vi "SFTP Error Status.vi"(8 "error in (no error)":errorcluster, 11 "return value":i32) -> (0 "error out":errorcluster, 3 "return value out":i32)   [LabVIEW 2017, in "libssh2.lvlib"]
uses:
  libssh2.lvlib
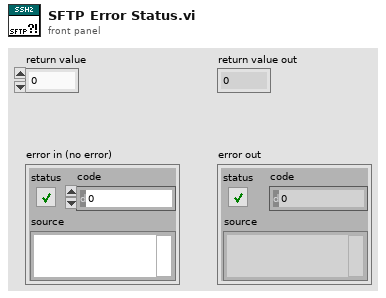
[diagram p1: front panel]
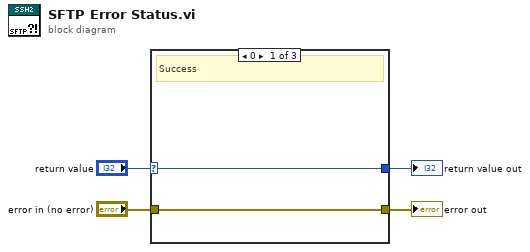
[diagram p0: block diagram]
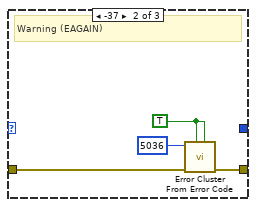
[diagram p2: hidden frame]
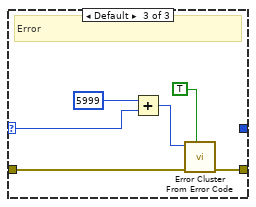
[diagram p3: hidden frame]
diagram:
  n1 = case shown="0" "return value" {
    selector: "return value" -> [w5 _ w11]
    tunnel: "error in (no error)" -> [w6 w10 w15]
    tunnel: [w6 w9 w14] -> w2
    tunnel: [w5 _ _] -> w1
    frame 0 {
      # "Success"
    }
    frame -37 {
      w7 = TRUE ("show call chain? (False)")
      # "Warning (EAGAIN)"
      n2 = call <vilib>:"Error Cluster From Error Code.vi"("is warning? (False)"=w7, "show call chain? (False)"=w7, "error in (no error)"=w10, "error code (0)"=5036) -> ("error out"=w9:errorcluster)  [unwired: 5 in]
    }
    frame Default {
      # "Error"
      n3 = Add(x=5999 ("return value"), y=w11) -> (x+y=w13:i32)
      n4 = call <vilib>:"Error Cluster From Error Code.vi"("show call chain? (False)"=TRUE, "error in (no error)"=w15, "error code (0)"=w13) -> ("error out"=w14:errorcluster)  [unwired: 6 in]
    }
  }
  "error out" <- w2
  "return value out" <- w1
